vi "Test XY Scanning with Alazar.vi"() -> ()   [LabVIEW 2018]
uses:
  Hardware Mfg/AlazarTech SDK/Controls/Alazar Engine Actions.ctl
  <vilib>/ErrorRing/Error Ring.xnode
  General/Controls/Queue Manager Actions.ctl
  General/Controls/data manager action.ctl
  General/Controls/Optical Parameters.ctl
  General/Controls/Vibratome Parameters.ctl
  General/Controls/Translation Stage Types.ctl
  Hardware Mfg/Thorlabs Translation Stages/Controls/Translation Stage Cluster.ctl
  General/Controls/Translation Stage Parameters.ctl
  General/Controls/Scan Direction.ctl
  General/Controls/Imaging Parameters.ctl
  General/Controls/System Parameters.ctl
  Hardware Mfg/AlazarTech SDK/Controls/Clock Controls.ctl
  Hardware Mfg/AlazarTech SDK/Controls/Alazar Device ID.ctl
  Hardware Mfg/AlazarTech SDK/Controls/Channel Input Controls.ctl
  Hardware Mfg/AlazarTech SDK/Controls/Trigger Engine Controls.ctl
  Hardware Mfg/AlazarTech SDK/Controls/General Trigger Settings.ctl
  Hardware Mfg/AlazarTech SDK/Controls/Alazar Acquisition Settings.ctl
  General/type defines/file type.ctl
  General/Controls/Control cluster.ctl
  General/type defines/Galvo parameters.ctl
  General/type defines/Alazar parameters.ctl
panel:
  out "# elements in data queue":i32
  out "# elements in display queue":i32
  out "time for 1 B-line":dbl
  out "# save":i32
  out "# display":i32
  in  "save?":bool
  out "Image":T1(plugin-control)
  out "error out":errorcluster
  in  "Alazar parameters":T2={"Trigger Settings"={"General Trigger Settings"={"Trigger Operation"=0, "Coupling ID"=2, "Range ID"=2, "Delay"=0, "Timeout Ticks"=0, "Mode"=1, "Parameter"=1}, "Trigger Engine 1"={"Trigger Engine"=0, "Source"=2, "Slope"=1, "Level"=140}, "Trigger Engine 2"={"Trigger Engine"=1, "Source"=3, "Slope"=1, "Level"=140}}, "Capture Clock"={"Sample Rate"=100, "Decimation"=0, "Source"=2, "Edge"=0}, "Device ID"={"System ID"=1, "Board ID"=1}, "Ch A Input Control"={"Channel"=1, "Coupling"=2, "Range"=10, "Impedance"=2}, "Ch B Input Control"={"Channel"=2, "Coupling"=2, "Range"=10, "Impedance"=2}, "Acq Settings"={"Window Type"=1, "Record Length"=1440, "Footer"=0, "Output Format"=11, "Offset"=0, "Records Per Buffer"=2048, "Samples per record"=2048, "Records Count (Records/Acq)"=2147483647}, "Cluster"={"FFT value magnification"=1000.0, "max queue size (-1, unlimited)"=-1, "File Type"=enum."Tiff", "file path"=path "C:/Users/BoasLab/Documents/Data/Alazar data/B-line/data/test.tif", "#A-lines to save"=2048, "#Z pixels to save"=100, "ImageDescription"="", "Convert to U16?"=FALSE}} {"Cluster"."FFT value magnification" min=0.0 max=10000.0 step=0.001 format="%.4f"; "Acq Settings"."Window Type" items=["DSP_WINDOW_NONE", "DSP_WINDOW_HANNING", "DSP_WINDOW_HAMMING", "DSP_WINDOW_BLACKMAN", "DSP_WINDOW_BLACKMAN_HARRIS", "DSP_WINDOW_BARTLETT"]; "Acq Settings"."Footer" items=["FOOTER_NONE", "FOOTER_NPT"]; "Acq Settings"."Output Format" items=["FLOAT_AMP2"=10, "FLOAT_LOG"=11]; "Ch B Input Control"."Channel" items=["A"=1, "B"=2, "C"=4, "D"=8]; "Ch B Input Control"."Coupling" items=["AC"=1, "DC"=2]; "Ch B Input Control"."Range" items=["20 mV"=1, "40 mV"=2, "50 mV"=3, "80 mV"=4, "100 mV"=5, "200 mV"=6, "400 mV"=7, "500 mV"=8, "800 mV"=9, "1 V"=10, "1.25 V"=33, "2 V"=11, "4 V"=12, "5 V"=13, "8 V"=14, "10 V"=15, "20 V"=16]; "Ch B Input Control"."Impedance" items=["1 MOhm"=1, "50 Ohm"=2, ""=0]; "Ch A Input Control"."Channel" items=["A"=1, "B"=2, "C"=4, "D"=8]; "Ch A Input Control"."Coupling" items=["AC"=1, "DC"=2]; "Ch A Input Control"."Range" items=["20 mV"=1, "40 mV"=2, "50 mV"=3, "80 mV"=4, "100 mV"=5, "200 mV"=6, "400 mV"=7, "500 mV"=8, "800 mV"=9, "1 V"=10, "1.25 V"=33, "2 V"=11, "4 V"=12, "5 V"=13, "8 V"=14, "10 V"=15, "20 V"=16]; "Ch A Input Control"."Impedance" items=["1 MOhm"=1, "50 Ohm"=2, ""=0]; "Capture Clock"."Edge" items=["Rising", "Falling"]; "Capture Clock"."Source" items=["Internal"=1, "Fast External"=2, "Medium External"=3, "Slow External"=4, "External AC"=5, "External DC"=6, "External 10MHz"=7]; "Trigger Settings"."General Trigger Settings"."Trigger Operation" items=["J", "K", "J OR K", "J AND K", "J XOR K", "J AND NOT K", "NOT J AND K"]; "Trigger Settings"."General Trigger Settings"."Coupling ID" items=["AC"=1, "DC"=2]; "Trigger Settings"."General Trigger Settings"."Range ID" items=["5 V", "1 V", "TTL"]; "Trigger Settings"."Trigger Engine 1"."Trigger Engine" items=["J", "K"]; "Trigger Settings"."Trigger Engine 1"."Source" items=["A", "B", "External", "Disable", "C", "D"]; "Trigger Settings"."Trigger Engine 1"."Slope" items=["Positive"=1, "Negative"=2]; "Trigger Settings"."Trigger Engine 2"."Trigger Engine" items=["J", "K"]; "Trigger Settings"."Trigger Engine 2"."Source" items=["A", "B", "External", "Disable", "C", "D"]; "Trigger Settings"."Trigger Engine 2"."Slope" items=["Positive"=1, "Negative"=2]}
  out "Acquisition":i32
  in  "stop":bool
  in  "Galvo HW Parameters":T11={"System Parameters"={"Optical Parameters"={"Obj. Focal Length [mm]"=45.0, "Scan Lens EFL[mm]"=59.5, "Tube Lens EFL[mm]"=205.0, "Galvo V Range (+/-)"=10.0, "Galvo Max Half Angle [Deg]"=19.0, "Max Galvo Range[%]"=0.0}, "Vibratome"={"Z Bottom [mm]"=0.0, "Pre Cut Dwell [s]"=0.0, "Blade Frequency [RPM]"=0, "Slice Speed [mm/s]"=0.0, "Post Cut Dwell [s]"=0.0, "Ramp Time [s]"=0.0, "Start X [mm]"=0.0, "Start Y [mm]"=0.0, "Slice Length [mm]"=0.0, "Slice Axis"=enum."Y Axis", "Controller VISA Ref"="COM4"}, "Table Stages"={"X Stage"={"Position"=0.0, "Is.Enabled?"=FALSE, "Is.Connected?"=FALSE, "Device SN"="45876539", "AccelerationMaximum"=0.0, "VelocityMaximum"=0.0, "Acceleration"=0.0, "Velocity"=0.0, "waitTimeout (ms)"=0, "Model"=enum."None", "Is.Homed?"=FALSE}, "Y Stage"={"Position"=0.0, "Is.Enabled?"=FALSE, "Is.Connected?"=FALSE, "Device SN"="45876539", "AccelerationMaximum"=0.0, "VelocityMaximum"=0.0, "Acceleration"=0.0, "Velocity"=0.0, "waitTimeout (ms)"=0, "Model"=enum."None", "Is.Homed?"=FALSE}, "Z Stage"={"Position"=0.0, "Is.Enabled?"=FALSE, "Is.Connected?"=FALSE, "Device SN"="45876539", "AccelerationMaximum"=0.0, "VelocityMaximum"=0.0, "Acceleration"=0.0, "Velocity"=0.0, "waitTimeout (ms)"=0, "Model"=enum."None", "Is.Homed?"=FALSE}}, "Imaging Parameter"={"Raster Scan Direction"=enum."Uni Directional", "Pixel Dwell Time [Clock Cycles]"=1, "Flyback Time [Clock Cycles]"=200, "XY Center [um]"={"X"=1.0, "Y"=1.0}, "Pixel Step Size [um]"=2.5, "XY Image Size"=enum."2048 x 2048", "Custom"=FALSE, "Custom Size"={"X"=10, "Y"=10}, "Line Averages"=1}, "Galvo HW Parameters"={"Analog Out Channel"="GalvoCtrl/ao0,GalvoCtrl/ao1", "Min Voltage"=-10.0, "Max Voltage"=10.0, "Pixel Clock Source"="/GalvoCtrl/PFI0", "Sample Rate"=1000.0, "Line Clock Out Ch"="GalvoCtrl/port0/line0"}, "Alazar parameters"={"Trigger Settings"={"General Trigger Settings"={"Trigger Operation"=0, "Coupling ID"=2, "Range ID"=2, "Delay"=0, "Timeout Ticks"=0, "Mode"=1, "Parameter"=1}, "Trigger Engine 1"={"Trigger Engine"=0, "Source"=2, "Slope"=1, "Level"=140}, "Trigger Engine 2"={"Trigger Engine"=1, "Source"=3, "Slope"=1, "Level"=140}}, "Capture Clock"={"Sample Rate"=100, "Decimation"=0, "Source"=2, "Edge"=0}, "Device ID"={"System ID"=1, "Board ID"=1}, "Ch A Input Control"={"Channel"=1, "Coupling"=2, "Range"=10, "Impedance"=2}, "Ch B Input Control"={"Channel"=2, "Coupling"=2, "Range"=10, "Impedance"=2}, "Acq Settings"={"Window Type"=1, "Record Length"=1440, "Footer"=0, "Output Format"=10, "Offset"=0, "Records Per Buffer"=2048, "Samples per record"=2048, "Records Count (Records/Acq)"=2147483647}, "Cluster"={"FFT value magnification"=1000.0, "max queue size (-1, unlimited)"=-1, "File Type"=enum."Tiff", "file path"=path "C:/Users/BoasLab/Documents/Data/Alazar data/B-line/data/test.tif", "#A-lines to save"=2048, "#Z pixels to save"=2048, "ImageDescription"="", "Convert to U16?"=FALSE}}, "Mosaic Paramter"={"X Axis"={"Start [mm]"=0.0, "Steps [pts]"=0, "End [mm]"=0.0}, "Y Axis"={"Start [mm]"=0.0, "Steps [pts]"=0, "End [mm]"=0.0}, "Scan Pattern"=enum."Uni-directional", "Overlap Options"={"Overlap Type"=enum."No Overlap", "Percent Overlap"=0, "Justify"=enum."Start"}}}} {"System Parameters"."Alazar parameters"."Cluster"."FFT value magnification" min=0.0 max=10000.0 step=0.001 format="%.4f"; "System Parameters"."Alazar parameters"."Acq Settings"."Window Type" items=["DSP_WINDOW_NONE", "DSP_WINDOW_HANNING", "DSP_WINDOW_HAMMING", "DSP_WINDOW_BLACKMAN", "DSP_WINDOW_BLACKMAN_HARRIS", "DSP_WINDOW_BARTLETT"]; "System Parameters"."Alazar parameters"."Acq Settings"."Footer" items=["FOOTER_NONE", "FOOTER_NPT"]; "System Parameters"."Alazar parameters"."Acq Settings"."Output Format" items=["FLOAT_AMP2"=10, "FLOAT_LOG"=11]; "System Parameters"."Alazar parameters"."Ch B Input Control"."Channel" items=["A"=1, "B"=2, "C"=4, "D"=8]; "System Parameters"."Alazar parameters"."Ch B Input Control"."Coupling" items=["AC"=1, "DC"=2]; "System Parameters"."Alazar parameters"."Ch B Input Control"."Range" items=["20 mV"=1, "40 mV"=2, "50 mV"=3, "80 mV"=4, "100 mV"=5, "200 mV"=6, "400 mV"=7, "500 mV"=8, "800 mV"=9, "1 V"=10, "1.25 V"=33, "2 V"=11, "4 V"=12, "5 V"=13, "8 V"=14, "10 V"=15, "20 V"=16]; "System Parameters"."Alazar parameters"."Ch B Input Control"."Impedance" items=["1 MOhm"=1, "50 Ohm"=2, ""=0]; "System Parameters"."Alazar parameters"."Ch A Input Control"."Channel" items=["A"=1, "B"=2, "C"=4, "D"=8]; "System Parameters"."Alazar parameters"."Ch A Input Control"."Coupling" items=["AC"=1, "DC"=2]; "System Parameters"."Alazar parameters"."Ch A Input Control"."Range" items=["20 mV"=1, "40 mV"=2, "50 mV"=3, "80 mV"=4, "100 mV"=5, "200 mV"=6, "400 mV"=7, "500 mV"=8, "800 mV"=9, "1 V"=10, "1.25 V"=33, "2 V"=11, "4 V"=12, "5 V"=13, "8 V"=14, "10 V"=15, "20 V"=16]; "System Parameters"."Alazar parameters"."Ch A Input Control"."Impedance" items=["1 MOhm"=1, "50 Ohm"=2, ""=0]; "System Parameters"."Alazar parameters"."Capture Clock"."Edge" items=["Rising", "Falling"]; "System Parameters"."Alazar parameters"."Capture Clock"."Source" items=["Internal"=1, "Fast External"=2, "Medium External"=3, "Slow External"=4, "External AC"=5, "External DC"=6, "External 10MHz"=7]; "System Parameters"."Alazar parameters"."Trigger Settings"."General Trigger Settings"."Trigger Operation" items=["J", "K", "J OR K", "J AND K", "J XOR K", "J AND NOT K", "NOT J AND K"]; "System Parameters"."Alazar parameters"."Trigger Settings"."General Trigger Settings"."Coupling ID" items=["AC"=1, "DC"=2]; "System Parameters"."Alazar parameters"."Trigger Settings"."General Trigger Settings"."Range ID" items=["5 V", "1 V", "TTL"]; "System Parameters"."Alazar parameters"."Trigger Settings"."Trigger Engine 1"."Trigger Engine" items=["J", "K"]; "System Parameters"."Alazar parameters"."Trigger Settings"."Trigger Engine 1"."Source" items=["A", "B", "External", "Disable", "C", "D"]; "System Parameters"."Alazar parameters"."Trigger Settings"."Trigger Engine 1"."Slope" items=["Positive"=1, "Negative"=2]; "System Parameters"."Alazar parameters"."Trigger Settings"."Trigger Engine 2"."Trigger Engine" items=["J", "K"]; "System Parameters"."Alazar parameters"."Trigger Settings"."Trigger Engine 2"."Source" items=["A", "B", "External", "Disable", "C", "D"]; "System Parameters"."Alazar parameters"."Trigger Settings"."Trigger Engine 2"."Slope" items=["Positive"=1, "Negative"=2]; "System Parameters"."Imaging Parameter"."Line Averages" min=1 max=30 step=1; "System Parameters"."Imaging Parameter"."Flyback Time [Clock Cycles]" max=10 step=1; "System Parameters"."Imaging Parameter"."Pixel Step Size [um]" min=0.0 max=10.0 step=0.01; "System Parameters"."Imaging Parameter"."Custom Size"."Y" min=1 max=30 step=1; "System Parameters"."Imaging Parameter"."Custom Size"."X" min=1 max=30 step=1; "System Parameters"."Imaging Parameter"."XY Center [um]"."Y" min=1.0 max=30.0 step=1.0; "System Parameters"."Imaging Parameter"."XY Center [um]"."X" min=1.0 max=30.0 step=1.0; "System Parameters"."Imaging Parameter"."Pixel Dwell Time [Clock Cycles]" max=10 step=1}
  # "X"
  # "X"
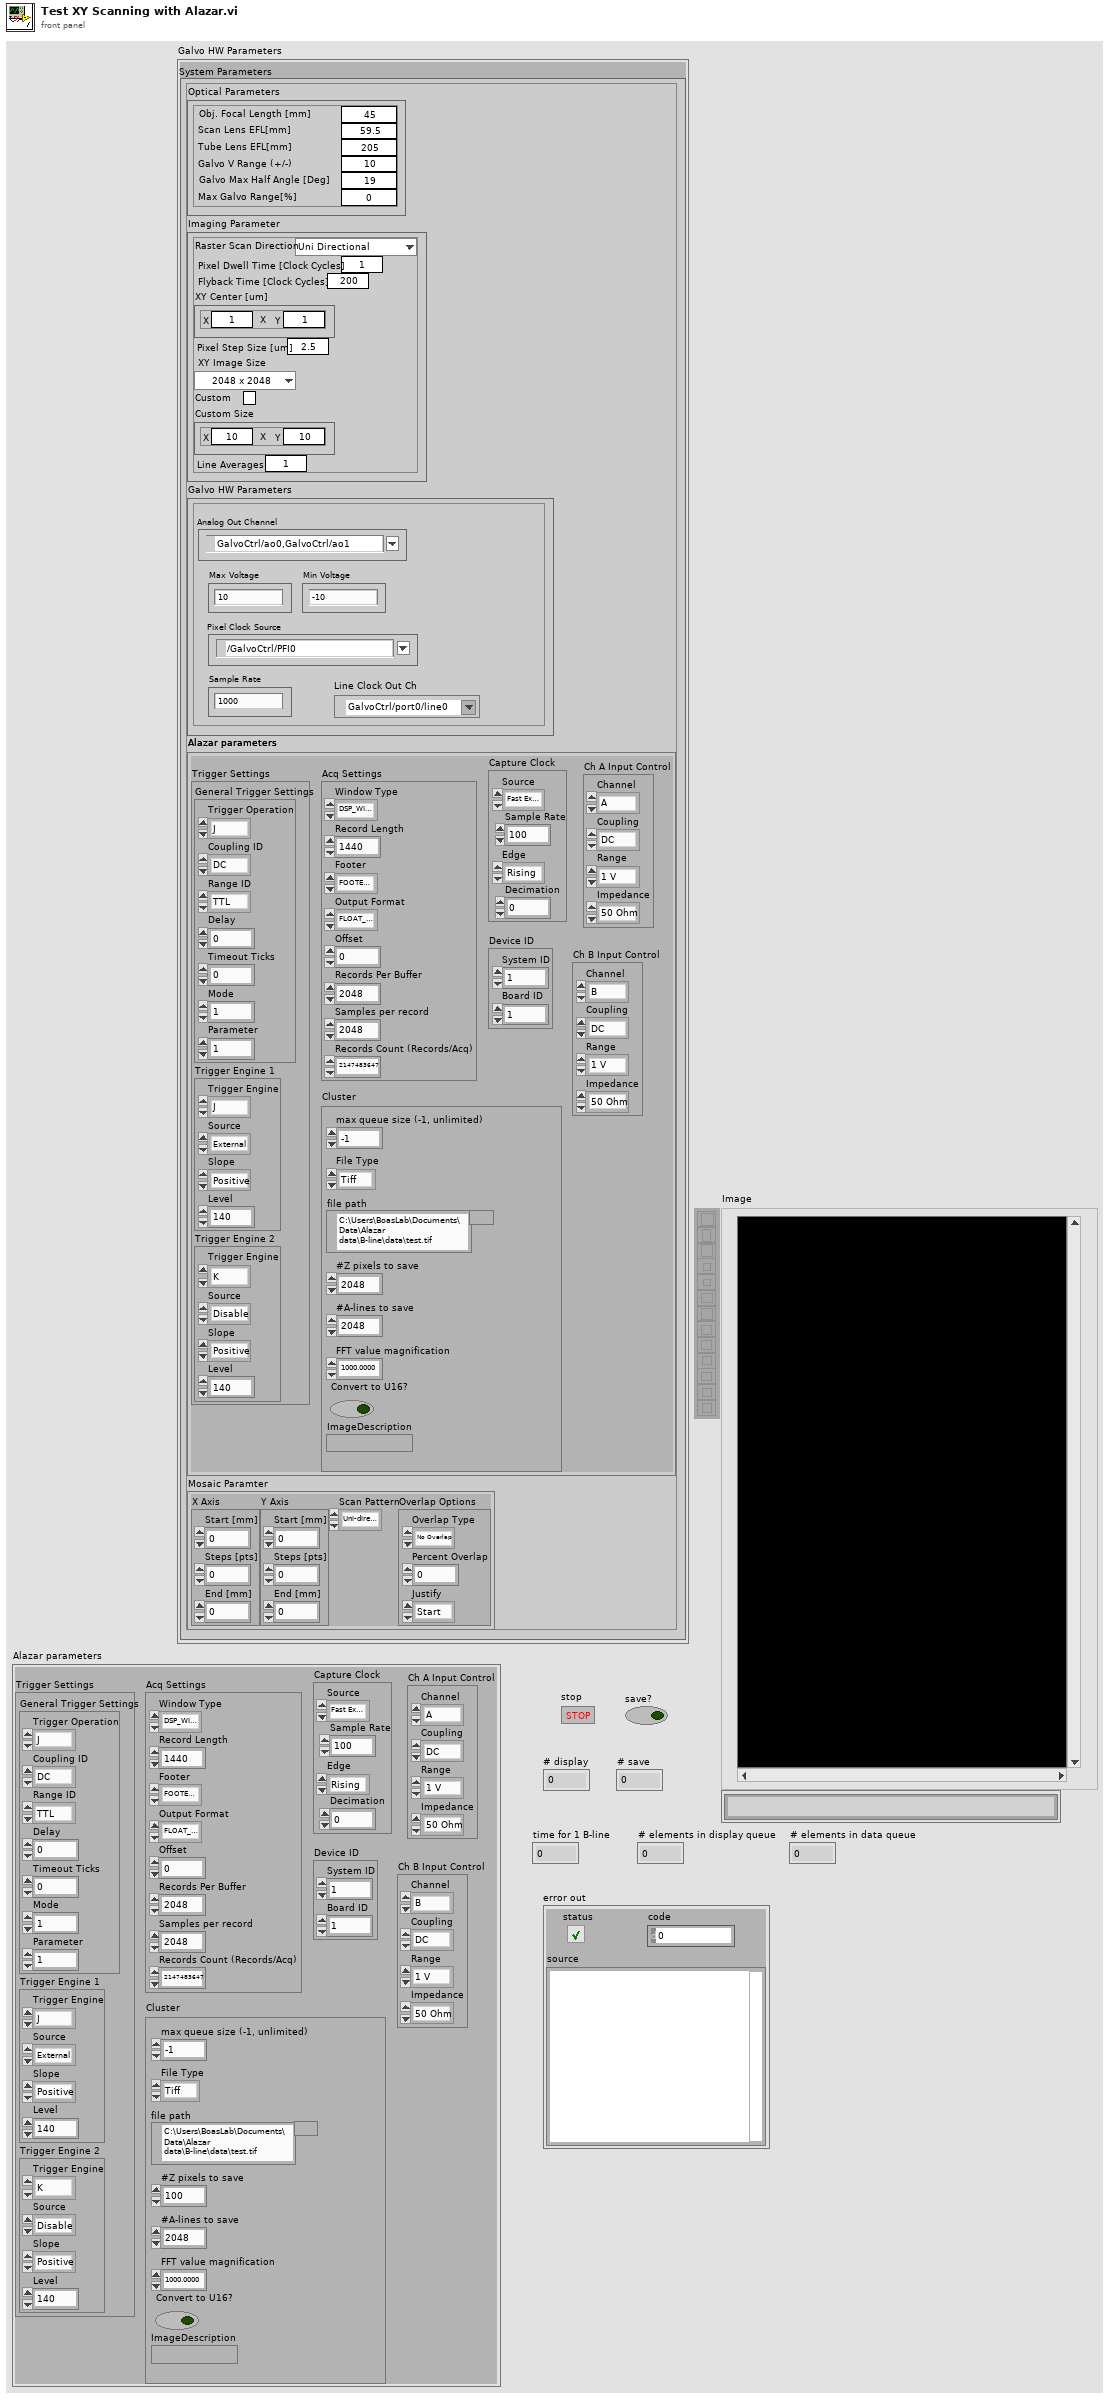
[diagram p1: front panel]
types:
  T1 = typedef "IMAQ Image.ctl" = refnum<image>
  T2 = typedef "Alazar parameters.ctl" = cluster{"Trigger Settings":cluster{"General Trigger Settings":T3, "Trigger Engine 1":T4, "Trigger Engine 2":T4}, "Capture Clock":T5, "Device ID":T6, "Ch A Input Control":T7, "Ch B Input Control":T7, "Acq Settings":T8, "Cluster":T9}
  T3 = typedef "General Trigger Settings.ctl" = cluster{"Trigger Operation":u32, "Coupling ID":u32, "Range ID":u32, "Delay":u32, "Timeout Ticks":u32, "Mode":u32, "Parameter":u32}
  T4 = typedef "Trigger Engine Controls.ctl" = cluster{"Trigger Engine":u32, "Source":u32, "Slope":u32, "Level":u32}
  T5 = typedef "Clock Controls.ctl" = cluster{"Sample Rate":u32, "Decimation":u32, "Source":u32, "Edge":u32}
  T6 = typedef "Alazar Device ID.ctl" = cluster{"System ID":u32, "Board ID":u32}
  T7 = typedef "Channel Input Controls.ctl" = cluster{"Channel":u8, "Coupling":u32, "Range":u32, "Impedance":u32}
  T8 = typedef "Alazar Acquisition Settings.ctl" = cluster{"Window Type":u32, "Record Length":u32, "Footer":u32, "Output Format":u32, "Offset":u32, "Records Per Buffer":u32, "Samples per record":u32, "Records Count (Records/Acq)":u32}
  T9 = typedef "Control cluster.ctl" = cluster{"FFT value magnification":dbl, "max queue size (-1, unlimited)":i32, "File Type":T10, "file path":path, "#A-lines to save":u32, "#Z pixels to save":u32, "ImageDescription":string, "Convert to U16?":bool}
  T10 = typedef "file type.ctl" = enum16{"text", "Tiff", "binary"}
  T11 = typedef "Galvo parameters.ctl" = cluster{"System Parameters":T12}
  T12 = typedef "System Parameters.ctl" = cluster{"Optical Parameters":T13, "Vibratome":T14, "Table Stages":T15, "Imaging Parameter":T18, "Galvo HW Parameters":cluster{"Analog Out Channel":tag, "Min Voltage":dbl, "Max Voltage":dbl, "Pixel Clock Source":tag, "Sample Rate":dbl, "Line Clock Out Ch":tag}, "Alazar parameters":T2, "Mosaic Paramter":cluster{"X Axis":cluster{"Start [mm]":dbl, "Steps [pts]":u16, "End [mm]":dbl}, "Y Axis":cluster{"Start [mm]":dbl, "Steps [pts]":u16, "End [mm]":dbl}, "Scan Pattern":enum16{"Uni-directional", "Bi-Directional", "Spiral Out", "Spiral In"}, "Overlap Options":cluster{"Overlap Type":enum16{"No Overlap", "X Only", "Y Only", "X and Y"}, "Percent Overlap":u8, "Justify":enum16{"Start", "Center", "End"}}}}
  T13 = typedef "Optical Parameters.ctl" = cluster{"Obj. Focal Length [mm]":dbl, "Scan Lens EFL[mm]":dbl, "Tube Lens EFL[mm]":dbl, "Galvo V Range (+/-)":dbl, "Galvo Max Half Angle [Deg]":dbl, "Max Galvo Range[%]":dbl}
  T14 = typedef "Vibratome Parameters.ctl" = cluster{"Z Bottom [mm]":dbl, "Pre Cut Dwell [s]":dbl, "Blade Frequency [RPM]":u16, "Slice Speed [mm/s]":dbl, "Post Cut Dwell [s]":dbl, "Ramp Time [s]":dbl, "Start X [mm]":dbl, "Start Y [mm]":dbl, "Slice Length [mm]":dbl, "Slice Axis":enum16{"X Axis", "Y Axis", "Z Axis"}, "Controller VISA Ref":refnum<visa-resource-name>}
  T15 = typedef "Translation Stage Parameters.ctl" = cluster{"X Stage":T16, "Y Stage":T16, "Z Stage":T16}
  T16 = typedef "Translation Stage Cluster.ctl" = cluster{"Position":dbl, "Is.Enabled?":bool, "Is.Connected?":bool, "Device SN":string, "AccelerationMaximum":dbl, "VelocityMaximum":dbl, "Acceleration":dbl, "Velocity":dbl, "waitTimeout (ms)":i32, "Model":T17, "Is.Homed?":bool}
  T17 = typedef "Translation Stage Types.ctl" = enum16{"None", "Thorlabs LTS", "Thorlabs MLJ"}
  T18 = typedef "Imaging Parameters.ctl" = cluster{"Raster Scan Direction":T19, "Pixel Dwell Time [Clock Cycles]":u16, "Flyback Time [Clock Cycles]":u16, "XY Center [um]":cluster{"X":dbl, "Y":dbl}, "Pixel Step Size [um]":dbl, "XY Image Size":enum16{"32 x 32", "64 x 64", "128 x 128", "256 x 256", "512 x 512", "1024 x 1024", "2048 x 2048"}, "Custom":bool, "Custom Size":cluster{"X":u16, "Y":u16}, "Line Averages":u8}
  T19 = typedef "Scan Direction.ctl" = enum16{"Uni Directional", "Bi Directional", "None"}
  T20 = enum16{"Configure channels", "Write Scan Pattern", "Start Galvo Task", "Is Task Done?", "Stop Galvo", "Uninit", "Init: Calc scan pattern"}
  T21 = typedef "Queue Manager Actions.ctl" = enum16{"Init", "Enqueue", "Enqueue All", "Preview Queue", "Dequeue", "Get Status", "Flush Queue", "Flush All Queues", "Release All Queues", "Release Queue", "Enqueue at Opposite End"}
  T22 = typedef "Alazar Engine Actions.ctl" = enum16{"Init", "Config Clock", "Config Ch", "Config Trig", "Config Non-FFT Acq.", "Non-FFT Acquire", "Load background from Non-FFT buffer", "enable background subtrac", "disable background subtrac", "load background from file", "load background from elsewhere", "start acquire", "background subtraction", "Config Acq.", "Acquire", "UnInit"}
  T23 = cluster{"General Trigger Settings":T3, "Trigger Engine 1":T4, "Trigger Engine 2":T4}
  T24 = cluster{"Analog Out Channel":tag, "Min Voltage":dbl, "Max Voltage":dbl, "Pixel Clock Source":tag, "Sample Rate":dbl, "Line Clock Out Ch":tag}
  T25 = typedef "data manager action.ctl" = enum16{"Init: open file", "save", "save as text", "Uninit: close file"}
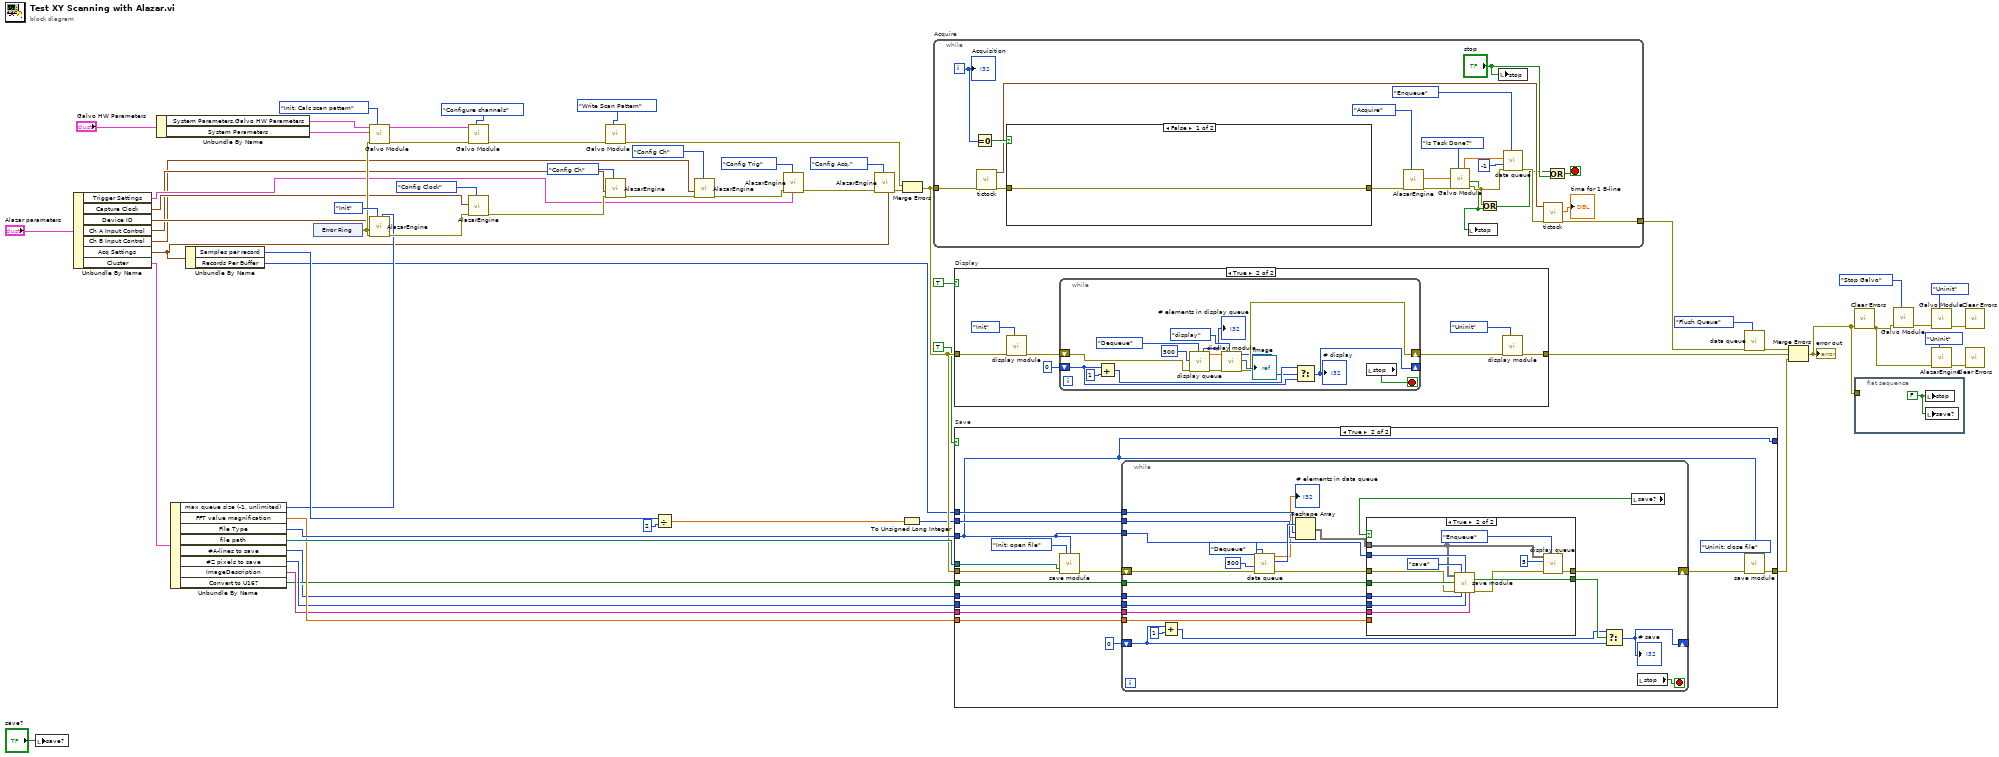
[diagram p0: block diagram]
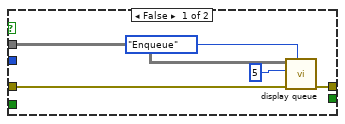
[diagram p3: hidden frame]
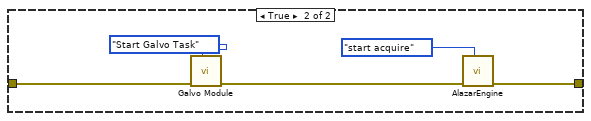
[diagram p5: hidden frame]
diagram:
  n1 = local write "save?"("save?") -> ()
  n2 = Unbundle By Name("Alazar parameters") -> ("Trigger Settings"=w14:T23, "Capture Clock"=w13:T5, "Device ID"=w12:T6, "Ch A Input Control"=w11:T7, "Ch B Input Control"=w10:T7, "Acq Settings"=w9:T8, "Cluster"=w8:T9)
  n3 = Unbundle By Name("Galvo HW Parameters") -> ("System Parameters.Galvo HW Parameters"=w16:T24, "System Parameters"=w17:T12)
  n4 = Unbundle By Name(w8) -> ("max queue size (-1, unlimited)"=w32:i32, "FFT value magnification"=w33:dbl, "File Type"=w37:T10, "file path"=w36:path, "#A-lines to save"=w24:u32, "#Z pixels to save"=w27:u32, "ImageDescription"=w26:string, "Convert to U16?"=w25:bool)
  n5 = Unbundle By Name(w9) -> ("Samples per record"=w40:u32, "Records Per Buffer"=w23:u32)
  n6 = xnode "Error Ring"() -> ("error out"=w21:errorcluster)
  n7 = call "Galvo Module.vi"("Action"=T20."Init: Calc scan pattern", "error in (no error)"=w21, "System Parameters"=w17) -> ("error out"=w20:errorcluster)  [unwired: 7 in, 1 out]
  n8 = call "AlazarEngine.vi"("Channel"=w32, "Action"=Alazar_Engine_Actions."Init", "error in (no error)"=w21, "Device ID"=w12) -> ("error out"=w59:errorcluster)  [unwired: 5 in, 2 out]
  n9 = call "Galvo Module.vi"("Action"=T20."Configure channels", "error in (no error)"=w20, 11:w16) -> ("error out"=w19:errorcluster)  [unwired: 7 in, 1 out]
  n10 = call "AlazarEngine.vi"("Action"=Alazar_Engine_Actions."Config Clock", "error in (no error)"=w59, "Capture Clock"=w13) -> ("error out"=w58:errorcluster)  [unwired: 6 in, 2 out]
  n11 = call "Galvo Module.vi"("Action"=T20."Write Scan Pattern", "error in (no error)"=w19) -> ("error out"=w60:errorcluster)  [unwired: 8 in, 1 out]
  n12 = call "AlazarEngine.vi"("Action"=Alazar_Engine_Actions."Config Ch", "error in (no error)"=w58, "Ch Input Control"=w11) -> ("error out"=w57:errorcluster)  [unwired: 6 in, 2 out]
  n13 = Divide(x=w40, y=u32 2) -> (x/y=w38:dbl)
  n14 = call "AlazarEngine.vi"("Action"=Alazar_Engine_Actions."Config Ch", "error in (no error)"=w57, "Ch Input Control"=w10) -> ("error out"=w52:errorcluster)  [unwired: 6 in, 2 out]
  n15 = call "AlazarEngine.vi"("Trigger Settings"=w14, "Action"=Alazar_Engine_Actions."Config Trig", "error in (no error)"=w52) -> ("error out"=w43:errorcluster)  [unwired: 6 in, 2 out]
  n16 = call "AlazarEngine.vi"("Acq Settings"=w9, "Action"=Alazar_Engine_Actions."Config Acq.", "error in (no error)"=w43) -> ("error out"=w49:errorcluster)  [unwired: 6 in, 2 out]
  n17 = To Unsigned Long Integer(number=w38) -> (unsigned 32bit integer=w22:u32)
  n18 = Merge Errors(w60, w49) -> (w31:errorcluster)
  n19 = while "Acquire" {
    tunnel: [w72] -> w44
    tunnel: w31 -> [w69]
    i -> [w77]
    stop <- w67 stop-if-true
    n20 = Equal To 0?(x=w77) -> (x = 0?=w80:bool)
    n21 = call "tictock.vi"("error in (no error)"=w69) -> ("error out"=w68:errorcluster, "seconds since 1Jan1904"=w70:timestamp)  [unwired: 8 in, 1 out]
    n22 = case shown="False" w80 {
      tunnel: [w81 w85] -> w79
      tunnel: w68 -> [w81 w84]
      frame False {
      }
      frame True {
        n23 = call "Galvo Module.vi"("Action"=T20."Start Galvo Task", "error in (no error)"=w84) -> ("error out"=w86:errorcluster)  [unwired: 8 in, 1 out]
        n24 = call "AlazarEngine.vi"("Action"=Alazar_Engine_Actions."start acquire", "error in (no error)"=w86) -> ("error out"=w85:errorcluster)  [unwired: 7 in, 2 out]
      }
    }
    n25 = call "AlazarEngine.vi"("Action"=Alazar_Engine_Actions."Acquire", "error in (no error)"=w79) -> ("error out"=w65:errorcluster, "Buffer"=w76:sgl[])  [unwired: 7 in, 1 out]
    n26 = call "Galvo Module.vi"("Action"=T20."Is Task Done?", "error in (no error)"=w65) -> ("error out"=w63:errorcluster, "task done?"=w61:bool)  [unwired: 8 in]
    n27 = local write "stop"(w61) -> ()
    n28 = Or(x=w63, y=w61) -> (x .or. y?=w62:bool)
    n29 = local write "stop"("stop") -> ()
    n30 = call "data queue.vi"("Action"=Queue_Manager_Actions."Enqueue", "error in (no error)"=w63, 9:-1 ("timeout in ms (-1)"), 10:w76) -> ("error out"=w73:errorcluster)  [unwired: 4 in, 3 out]
    n31 = call "tictock.vi"("error in (no error)"=w73, "seconds since 1Jan1904 2"=w70) -> ("error out"=w72:errorcluster, "Numeric"=→"time for 1 B-line":dbl)  [unwired: 7 in, 1 out]
    n32 = Or(x=w62, y="stop") -> (x .or. y?=w67:bool)
    "Acquisition" <- w77
  }
  n33 = case "Display" shown="True" TRUE {
    tunnel: [w87 w90] -> w35
    tunnel: w31 -> [w87 w89]
    frame False {
    }
    frame True {
      n34 = call "display module.vi"("FOV: #A-lines"=enum16{"Init", "display", "Uninit"}."Init" ("Action"), "error in"=w89) -> ("error out"=w93:errorcluster)  [unwired: 7 in, 2 out]
      n35 = while {
        shift-right: [w106] -> w91
        shift-left: w93 -> [w100]
        shift-right: [w101] -> _
        shift-left: 0 -> [w102]
        stop <- w109 stop-if-true
        n36 = Add(x=w102, y=1) -> (x+y=w104:i32)
        n37 = call "display queue.vi"("Action"=Queue_Manager_Actions."Dequeue", "error in (no error)"=w100, "time out"=500 ("timeout in ms (-1)")) -> ("error out"=w97:errorcluster, "output data"=w96:sgl[], "# elements in queue"=→"# elements in display queue":i32)  [unwired: 4 in, 2 out]
        n38 = call "display module.vi"("FOV: #A-lines"=enum16{"Init", "display", "Uninit"}."display" ("Action"), "error in"=w97, 11:w96) -> ("error out"=w106:errorcluster, "Image"=→"Image":T1, "elements in display queue"=w103:i32)  [unwired: 6 in]
        n39 = Select(t=w104, s=w103, f=w102) -> (s? t:f=w101:i32)
        "# display" <- w101
        n40 = local read "stop"() -> (w109:bool)
      }
      n41 = call "display module.vi"("FOV: #A-lines"=enum16{"Init", "display", "Uninit"}."Uninit" ("Action"), "error in"=w91) -> ("error out"=w90:errorcluster)  [unwired: 7 in, 2 out]
    }
  }
  n42 = case "Save" shown="True" TRUE {
    tunnel: w37 -> [_ w111]
    tunnel: w36 -> [_ w126]
    tunnel: [w110 w125] -> w34
    tunnel: w33 -> [_ w124]
    tunnel: w31 -> [w110 w123]
    tunnel: w27 -> [_ w119]
    tunnel: w26 -> [_ w116]
    tunnel: w25 -> [_ w117]
    tunnel: w24 -> [_ w118]
    tunnel: w22 -> [_ w115]
    tunnel: w23 -> [_ w114]
    tunnel: [_ w111] -> _
    frame False {
    }
    frame True {
      n43 = call "save module.vi"("action"=data_manager_action."Init: open file", "File Type"=w111, "file path and name"=w126, "error in (no error)"=w123) -> ("error out"=w122:errorcluster)  [unwired: 10 in, 1 out]
      n44 = while {
        tunnel: w124 -> [w148]
        shift-right: [w147] -> w121
        shift-left: w122 -> [w139]
        shift-right: [w142] -> _
        shift-left: 0 -> [w143]
        tunnel: w119 -> [w136]
        tunnel: w118 -> [w135]
        tunnel: w117 -> [w134]
        tunnel: w116 -> [w133]
        tunnel: w115 -> [w131]
        tunnel: w114 -> [w130]
        tunnel: w111 -> [w128]
        stop <- w149 stop-if-true
        n45 = Add(x=w143, y=1) -> (x+y=w144:i32)
        n46 = call "data queue.vi"("Action"=Queue_Manager_Actions."Dequeue", "error in (no error)"=w139, 9:500 ("timeout in ms (-1)")) -> ("error out"=w137:errorcluster, "# elements in queue"=w132:i32, "data out"=→"# elements in data queue":sgl[])  [unwired: 5 in, 1 out]
        n47 = Reshape Array(w132, w130, w131) -> (w129:void[][])
        n48 = local read "save?"() -> (w138:bool)
        n49 = case shown="True" w138 {
          tunnel: w148 -> [_ _]
          tunnel: [w153 w155] -> w147
          tunnel: [_ w167] -> w146
          tunnel: w137 -> [w154 w157]
          tunnel: w136 -> [_ w164]
          tunnel: w135 -> [_ w163]
          tunnel: w134 -> [_ w162]
          tunnel: w133 -> [_ w161]
          tunnel: w129 -> [w152 w158]
          tunnel: w128 -> [_ w159]
          frame False {
            n50 = call "display queue.vi"("Action"=Queue_Manager_Actions."Enqueue", "error in (no error)"=w154, "time out"=5, "input data"=w152) -> ("error out"=w153:errorcluster)  [unwired: 3 in, 4 out]
          }
          frame True {
            n51 = call "save module.vi"("data in"=w158, "action"=data_manager_action."save", "File Type"=w159, "Convert to U16?"=w162, "error in (no error)"=w157, "# A-lines to save"=w163, "#Z pixels to save"=w164, "ImageDescription"=w161) -> ("save successful?"=w167:bool, "error out"=w156:errorcluster)  [unwired: 6 in]
            n52 = call "display queue.vi"("Action"=Queue_Manager_Actions."Enqueue", "error in (no error)"=w156, "time out"=5, "input data"=w158) -> ("error out"=w155:errorcluster)  [unwired: 3 in, 4 out]
          }
        }
        n53 = Select(t=w144, s=w146, f=w143) -> (s? t:f=w142:i32)
        "# save" <- w142
        n54 = local read "stop"() -> (w149:bool)
      }
      n55 = call "save module.vi"("action"=data_manager_action."Uninit: close file", "File Type"=w111, "error in (no error)"=w121) -> ("error out"=w125:errorcluster)  [unwired: 11 in, 1 out]
    }
  }
  n56 = call "data queue.vi"("Action"=Queue_Manager_Actions."Flush Queue", "error in (no error)"=w44) -> ("error out"=w42:errorcluster)  [unwired: 6 in, 3 out]
  n57 = Merge Errors(w42, w35, w34) -> (w45:errorcluster)
  "error out" <- w45
  n58 = call <vilib>:"Clear Errors.vi"("error in (no error)"=w45) -> ("error out"=w3:errorcluster)  [unwired: 5 in, 1 out]
  n59 = flat-sequence {
    tunnel: w45 -> [_]
    frame #0 {
      w168 = FALSE ("stop")
      n60 = local write "stop"(w168) -> ()
      n61 = local write "save?"(w168) -> ()
    }
  }
  n62 = call "Galvo Module.vi"("Action"=T20."Stop Galvo", "error in (no error)"=w3) -> ("error out"=w2:errorcluster)  [unwired: 8 in, 1 out]
  n63 = call "Galvo Module.vi"("Action"=T20."Uninit", "error in (no error)"=w2) -> ("error out"=w47:errorcluster)  [unwired: 8 in, 1 out]
  n64 = call "AlazarEngine.vi"("Action"=Alazar_Engine_Actions."UnInit", "error in (no error)"=w3) -> ("error out"=w46:errorcluster)  [unwired: 7 in, 2 out]
  n65 = call <vilib>:"Clear Errors.vi"("error in (no error)"=w47) -> ()  [unwired: 5 in, 2 out]
  n66 = call <vilib>:"Clear Errors.vi"("error in (no error)"=w46) -> ()  [unwired: 5 in, 2 out]
